vi "Toolpath.vi"(4 "Dot Settings":refnum<class "Dot Settings.lvclass">[](array[class]), 5 "Path Settings":refnum<class "Path Settings.lvclass">[](array[class]), 6 "Funnel Properties":T3[](array[typedef]) {"Direction" items=["Forward", "Backward"]}, 7 "Parsing Data":T9, 8 "Path Properties":T7[](array[typedef]) {"Fill Orientation" items=["Horizontal", "Vertical", ""]; "Direction" items=["Forward", "Backward"]}, 9 "Rectangle Properties":T6[](array[typedef]) {"Fill Orientation" items=["Horizontal", "Vertical", ""]; "Direction" items=["Forward", "Backward"]}) -> (2 "Estimated Time Required":timestamp format="%<%I:%M:%S>T", 3 "Lithography Data":T2(array[cluster]))   [LabVIEW 2019]
uses:
  <vilib>/Analysis/Matrix/Datatypes/RealMatrix.ctl
  Classes/Parse/Dot/Dot.lvclass
  typedefs/Path Properties - cluster.ctl
  typedefs/Voltage - cluster.ctl
  typedefs/Schedule - enum.ctl
  <userlib>/LevyLab/Relay Box/Typedefs/Resistor--enum.ctl
  typedefs/Rectangle Properties - cluster.ctl
  typedefs/Funnel Properties - cluster.ctl
  Classes/Settings/Dot Settings/Dot Settings.lvclass
  Classes/Settings/Path Settings/Path Settings.lvclass
  <vilib>/Analysis/Matrix/NI_Matrix.lvlib
  <userlib>/LevyLab/Relay Box/Relay-Box.lvclass
panel:
  out "Dots":u32
  out "Rects":u32
  out "Funnels":u32
  out "Paths":u32
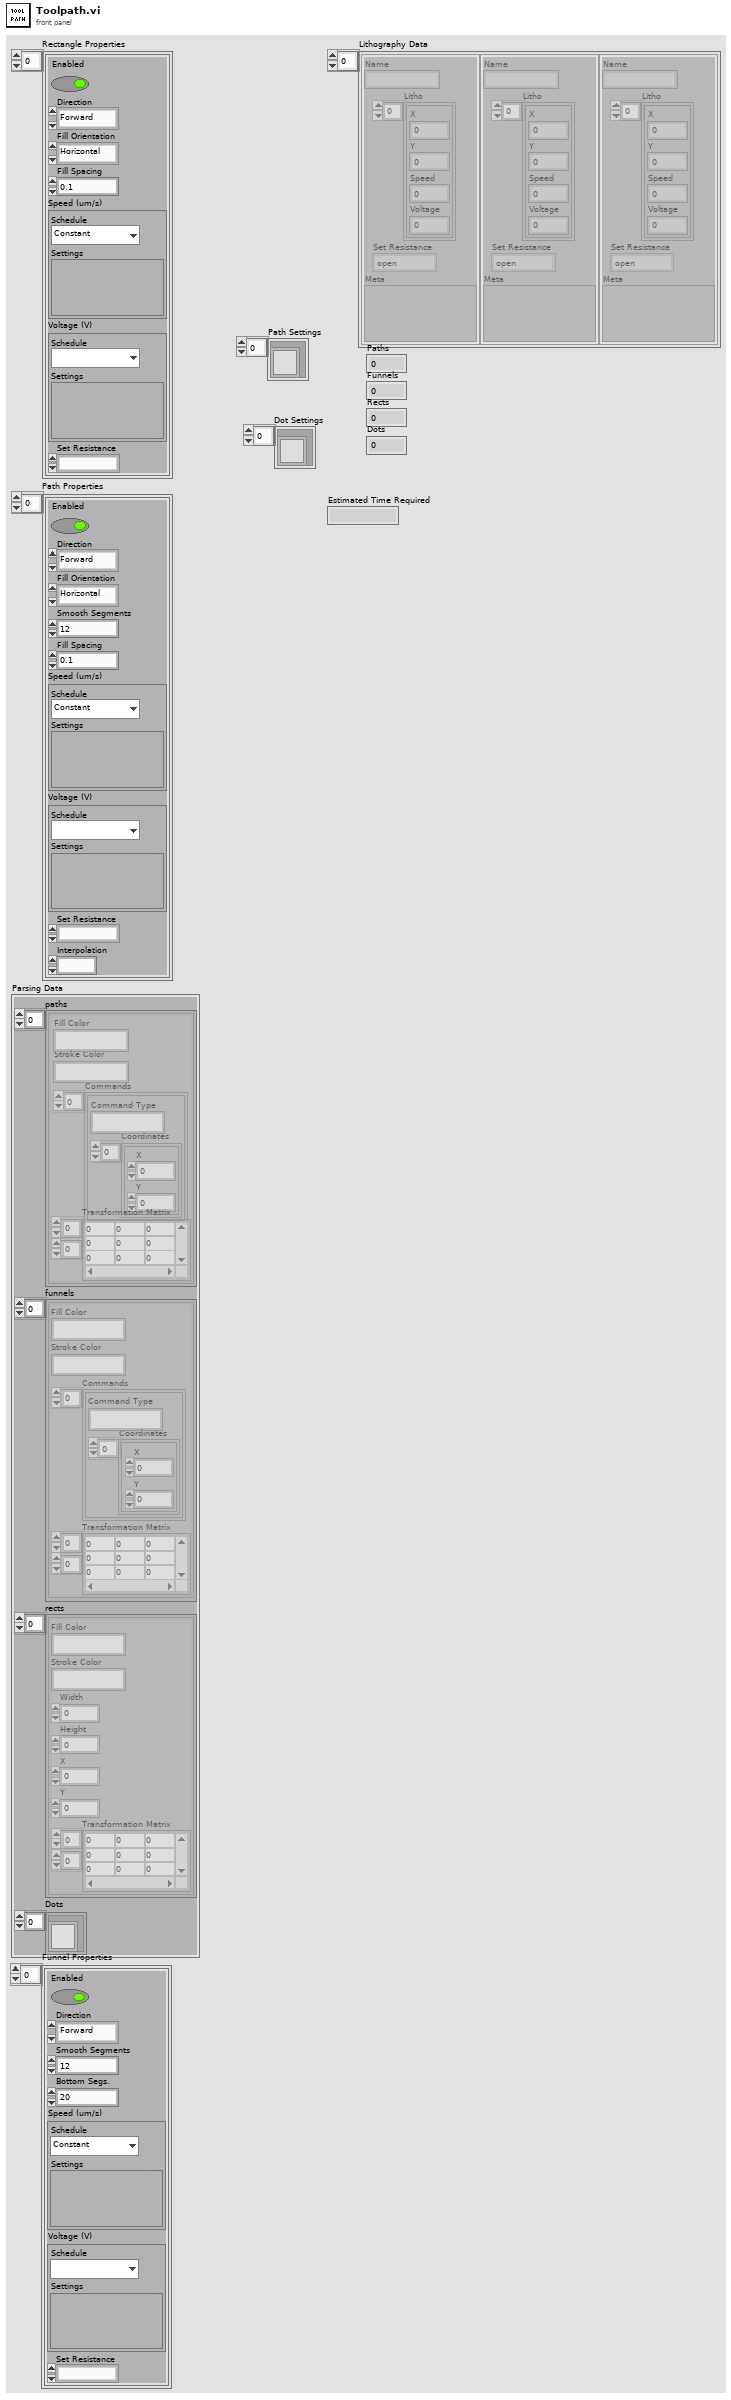
[diagram p1: front panel]
types:
  T1 = typedef "Relay-Box.lvclass/Resistor--enum.ctl" = enum16{"open", "discharge tip", "0 ohms", "100k ohm", "10M ohm", "1G ohm"}
  T2 = cluster{"Name":string, "Litho":cluster{"X":dbl, "Y":dbl, "Speed":dbl, "Voltage":dbl}[], "Set Resistance":T1, "Meta":variant}[]
  T3 = typedef "Funnel Properties - cluster.ctl" = cluster{"Enabled":bool, "Direction":u16, "Smooth Segments":dbl, "Bottom Segs.":dbl, "Speed (um/s)":T4, "Voltage (V)":T4, "Set Resistance":T1}
  T4 = typedef "Voltage - cluster.ctl" = cluster{"Schedule":T5, "Settings":variant}
  T5 = typedef "Schedule - enum.ctl" = enum16{"Constant", "Ramp", "Fn. Generator", "Formula"}
  T6 = typedef "Rectangle Properties - cluster.ctl" = cluster{"Enabled":bool, "Direction":u16, "Fill Orientation":u16, "Fill Spacing":dbl, "Speed (um/s)":T4, "Voltage (V)":T4, "Set Resistance":T1}
  T7 = typedef "Path Properties - cluster.ctl" = cluster{"Enabled":bool, "Direction":u16, "Fill Orientation":u16, "Smooth Segments":dbl, "Fill Spacing":dbl, "Speed (um/s)":T4, "Voltage (V)":T4, "Set Resistance":T1, "Interpolation":dbl}
  T8 = typedef "NI_Matrix.lvlib/RealMatrix.ctl" = dbl[][]
  T9 = cluster{"paths":cluster{"Fill Color":string, "Stroke Color":string, "Commands":cluster{"Command Type":string, "Coordinates":cluster{"X":dbl, "Y":dbl}[]}[], "Transformation Matrix":T8}[], "funnels":cluster{"Fill Color":string, "Stroke Color":string, "Commands":cluster{"Command Type":string, "Coordinates":cluster{"X":dbl, "Y":dbl}[]}[], "Transformation Matrix":T8}[], "rects":cluster{"Fill Color":string, "Stroke Color":string, "Width":dbl, "Height":dbl, "X":dbl, "Y":dbl, "Transformation Matrix":T8}[], "Dots":refnum<class "Dot.lvclass">[]}
  T10 = cluster{"Fill Color":string, "Stroke Color":string, "Commands":cluster{"Command Type":string, "Coordinates":cluster{"X":dbl, "Y":dbl}[]}[], "Transformation Matrix":T8}[]
  T11 = cluster{"Fill Color":string, "Stroke Color":string, "Width":dbl, "Height":dbl, "X":dbl, "Y":dbl, "Transformation Matrix":T8}[]
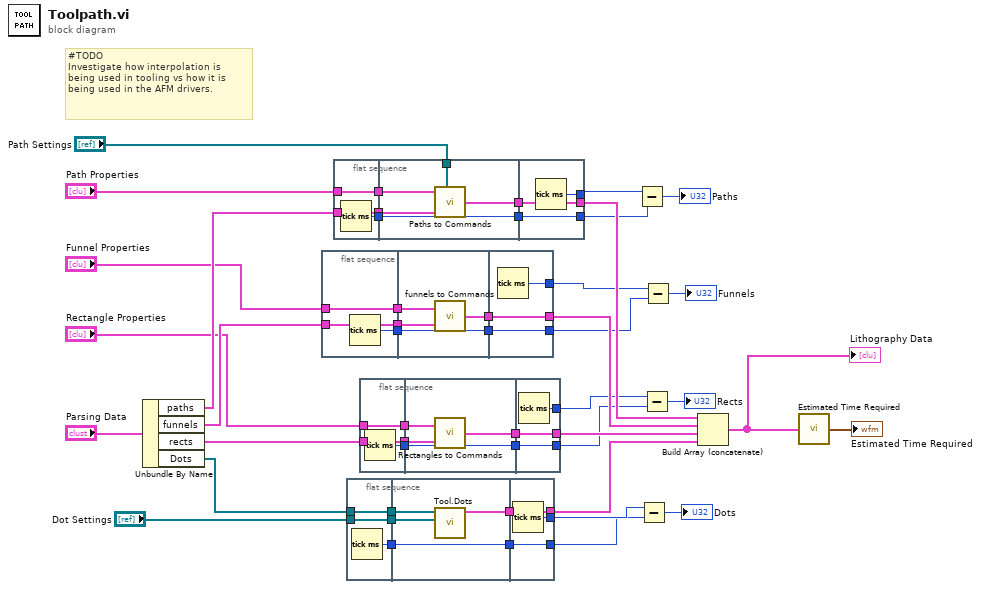
[diagram p0: block diagram]
diagram:
  # "#TODO\nInvestigate how interpolation is being used in tooling vs how it is being used in the AFM drivers."
  n1 = Unbundle By Name("Parsing Data") -> ("paths"=w48:T10, "funnels"=w47:T10, "rects"=w46:T11, "Dots"=w35:refnum<class "Dot.lvclass">[])
  n2 = flat-sequence {
    tunnel: "Funnel Properties" -> [w50]
    tunnel: w47 -> [w51]
    tunnel: [w51] -> w25
    tunnel: [w50] -> w24
    tunnel: [w49] -> w13
    tunnel: [w54] -> w26
    tunnel: w25 -> [w55]
    tunnel: w24 -> [w53]
    tunnel: [w52] -> w14
    tunnel: w13 -> [w52]
    tunnel: [w58] -> w44
    tunnel: w26 -> [w58]
    tunnel: [w57] -> w8
    tunnel: [w56] -> w7
    tunnel: w14 -> [w56]
    frame #0 {
      n3 = Tick Count (ms)() -> (millisecond timer value=w49:u32)
    }
    frame #1 {
      n4 = call "funnels to Commands.vi"("funnels"=w55, "Funnel Properties"=w53) -> ("Lithography Data"=w54:T2)
    }
    frame #2 {
      n5 = Tick Count (ms)() -> (millisecond timer value=w57:u32)
    }
  }
  n6 = flat-sequence {
    tunnel: "Path Properties" -> [w60]
    tunnel: w48 -> [w61]
    tunnel: [w61] -> w23
    tunnel: [w60] -> w22
    tunnel: [w59] -> w19
    tunnel: "Path Settings" -> [w63]
    tunnel: w23 -> [w66]
    tunnel: w22 -> [w65]
    tunnel: [w64] -> w21
    tunnel: [w62] -> w20
    tunnel: w19 -> [w62]
    tunnel: [w69] -> w39
    tunnel: w21 -> [w69]
    tunnel: [w68] -> w6
    tunnel: [w67] -> w5
    tunnel: w20 -> [w67]
    frame #0 {
      n7 = Tick Count (ms)() -> (millisecond timer value=w59:u32)
    }
    frame #1 {
      n8 = call "Paths to Commands.vi"("Path Properties"=w65, "Path Settings"=w63, "paths"=w66) -> ("Lithography Data"=w64:T2)  [unwired: 2 in]
    }
    frame #2 {
      n9 = Tick Count (ms)() -> (millisecond timer value=w68:u32)
    }
  }
  n10 = flat-sequence {
    tunnel: "Dot Settings" -> [w71]
    tunnel: w35 -> [w72]
    tunnel: [w72] -> w32
    tunnel: [w71] -> w31
    tunnel: [w70] -> w17
    tunnel: w32 -> [w75]
    tunnel: w31 -> [w74]
    tunnel: [w76] -> w30
    tunnel: [w73] -> w18
    tunnel: w17 -> [w73]
    tunnel: [w79] -> w36
    tunnel: w30 -> [w79]
    tunnel: [w78] -> w11
    tunnel: w18 -> [w78]
    tunnel: [w77] -> w12
    frame #0 {
      n11 = Tick Count (ms)() -> (millisecond timer value=w70:u32)
    }
    frame #1 {
      n12 = call "Tool.Dots.vi"("Dot Settings"=w74, "Dots"=w75) -> ("Commands"=w76:T2)  [unwired: 9 in]
    }
    frame #2 {
      n13 = Tick Count (ms)() -> (millisecond timer value=w77:u32)
    }
  }
  n14 = flat-sequence {
    tunnel: "Rectangle Properties" -> [w81]
    tunnel: w46 -> [w82]
    tunnel: [w82] -> w28
    tunnel: [w81] -> w27
    tunnel: [w80] -> w15
    tunnel: [w85] -> w29
    tunnel: w28 -> [w86]
    tunnel: w27 -> [w84]
    tunnel: [w83] -> w16
    tunnel: w15 -> [w83]
    tunnel: [w89] -> w43
    tunnel: w29 -> [w89]
    tunnel: [w88] -> w9
    tunnel: w16 -> [w88]
    tunnel: [w87] -> w10
    frame #0 {
      n15 = Tick Count (ms)() -> (millisecond timer value=w80:u32)
    }
    frame #1 {
      n16 = call "Rectangles to Commands.vi"("rects"=w86, "Rectangle Properties"=w84) -> ("Lithography Data"=w85:T2)
    }
    frame #2 {
      n17 = Tick Count (ms)() -> (millisecond timer value=w87:u32)
    }
  }
  n18 = Subtract(x=w6, y=w5) -> (x-y=→"Paths":u32)
  n19 = Subtract(x=w12, y=w11) -> (x-y=→"Dots":u32)
  n20 = Subtract(x=w10, y=w9) -> (x-y=→"Rects":u32)
  n21 = Subtract(x=w8, y=w7) -> (x-y=→"Funnels":u32)
  n22 = Build Array (concatenate)(w39, w44, w43, w36) -> (w37:T2)
  "Lithography Data" <- w37
  n23 = call "Estimated Time Required.vi"("Lithography Data"=w37) -> ("Estimated Time Required"=→"Estimated Time Required":timestamp)
